vi "Get_SubArray.vi"(9 "length":i32=4, 10 "index":i32, 11 "AO WF":waveform(dbl)[](array[waveform])) -> (3 "Sub array":waveform(dbl)[](array[waveform]))   [LabVIEW 2025]
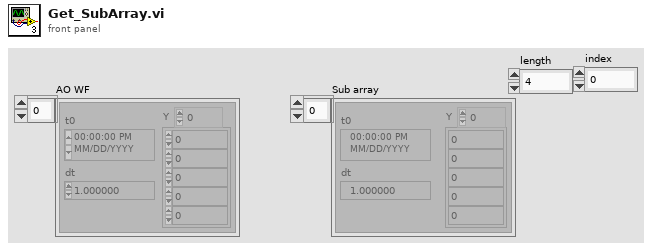
[diagram p1: front panel]
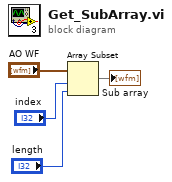
[diagram p0: block diagram]
diagram:
  n1 = Array Subset(array="AO WF", index="index", length="length") -> (→"Sub array":waveform(dbl)[])
